vi "Lec1.vi"() -> ()   [LabVIEW 2019]
panel:
  out "String 2":string
  in  "String":string
  out "Boolean 2":bool
  in  "Boolean":bool
  out "Numeric 3":dbl
  out "Gauge":dbl(knob) scale=0.0..10.0
  in  "Slide":dbl(slide) scale=0.0..10.0
  out "Numeric 2":dbl
  in  "Numeric":dbl
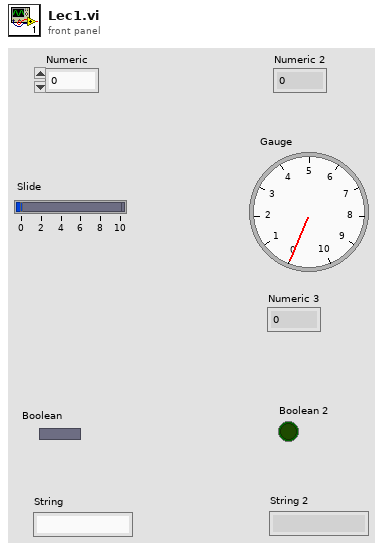
[diagram p1: front panel]
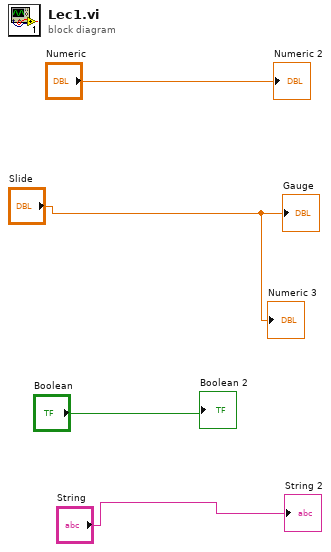
[diagram p0: block diagram]
diagram:
  "Numeric 2" <- "Numeric"
  "Gauge" <- "Slide"
  "Numeric 3" <- "Slide"
  "Boolean 2" <- "Boolean"
  "String 2" <- "String"
